vi "Speed Graph Window-Notifier.vi"(6 "ignore previous (F)":bool, 8 "error in":errorcluster, 9 "Timeout waiting in ms (-1)":i32=-1, 10 "Speed window data":T1, 11 "Notifier Function":T3=enum."Wait on notification") -> (0 "error out":errorcluster, 2 "Notification data received":T1, 3 "Timed out waiting":bool)   [LabVIEW 2013]
uses:
  Typedefs/Notifier Function.ctl
  Typedefs/Speed window notifier data.ctl
  Typedefs/Speed logging states enum.ctl
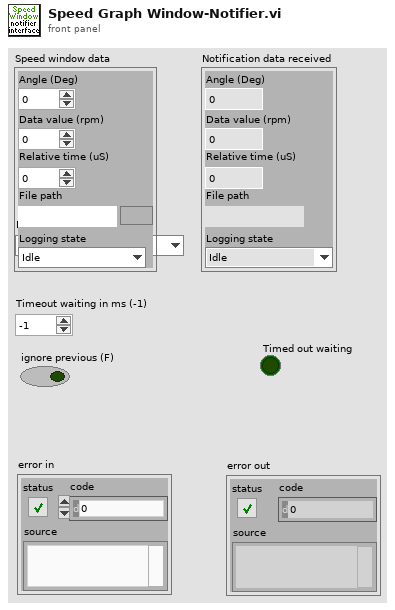
[diagram p1: front panel]
types:
  T1 = typedef "Speed window notifier data.ctl" = cluster{"Angle (Deg)":dbl, "Data value (rpm)":dbl, "Relative time (uS)":i32, "File path":path, "Logging state":T2}
  T2 = typedef "Speed logging states enum.ctl" = enum16{"Idle", "Open file", "Log", "Close file"}
  T3 = typedef "Notifier Function.ctl" = enum16{"Send notifier", "Wait on notification", "Release notifier"}
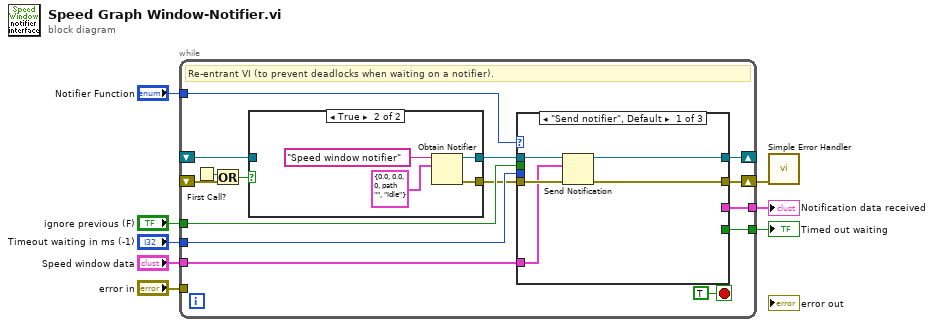
[diagram p0: block diagram]
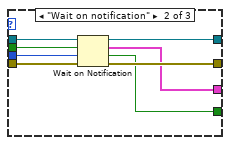
[diagram p2: hidden frame]
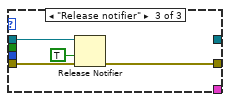
[diagram p3: hidden frame]
diagram:
  n1 = while {
    shift-right: [w20] -> _
    shift-left: _ -> [w22]
    tunnel: "Notifier Function" -> [w19]
    tunnel: "Timeout waiting in ms (-1)" -> [w18]
    tunnel: "ignore previous (F)" -> [w17]
    shift-right: [w15] -> w8
    shift-left: _ -> [w14]
    tunnel: [w11] -> w4
    tunnel: [w10] -> w2
    tunnel: "Speed window data" -> [w9]
    tunnel: "error in" -> [_]
    stop <- TRUE stop-if-true
    # "Re-entrant VI (to prevent deadlocks when waiting on a notifier)."
    n2 = First Call?() -> (First Call?: T/F=w13:bool)
    n3 = Or(x=w13, y=w14) -> (x .or. y?=w12:bool)
    n4 = case shown="True" w12 {
      tunnel: [w41 w44] -> w21
      tunnel: w22 -> [w41 _]
      tunnel: [_ w43] -> w16
      frame False {
      }
      frame True {
        n5 = Obtain Notifier(name (unnamed)="Speed window notifier", notification data type=T1 {"Angle (Deg)"=0.0, "Data value (rpm)"=0.0, "Relative time (uS)"=0, "File path"=path "", "Logging state"=enum."Idle"} ("Speed window data")) -> (notifier out=w44:refnum<notifier>, error out=w43:errorcluster)  [unwired: 2 in, 1 out]
      }
    }
    n6 = case shown="\"Send notifier\", Default" w19 {
      tunnel: w21 -> [w28 w34 w40]
      tunnel: [w27 w33 _] -> w20
      tunnel: w18 -> [_ w35 _]
      tunnel: w17 -> [_ w36 _]
      tunnel: w16 -> [w26 w31 w38]
      tunnel: [w25 w32 w39] -> w15
      tunnel: [_ w30 _] -> w11
      tunnel: [_ w29 _] -> w10
      tunnel: w9 -> [w24 _ _]
      frame "Send notifier", Default {
        n7 = Send Notification(notification=w24, notifier=w28, error in (no error)=w26) -> (notifier out=w27:refnum<notifier>, error out=w25:errorcluster)
      }
      frame "Wait on notification" {
        n8 = Wait on Notification(notifier=w34, ignore previous (F)=w36, timeout in ms (-1)=w35, error in (no error)=w31) -> (notifier out=w33:refnum<notifier>, notification=w29:T1, timed out?=w30:bool, error out=w32:errorcluster)
      }
      frame "Release notifier" {
        n9 = Release Notifier(notifier=w40, force destroy? (F)=TRUE, error in (no error)=w38) -> (error out=w39:errorcluster)  [unwired: 2 out]
      }
    }
  }
  "Timed out waiting" <- w4
  "Notification data received" <- w2
  n10 = call <vilib>:"Simple Error Handler.vi"("error in (no error)"=w8) -> ()  [unwired: 4 in, 5 out]
